vi "Launch Hardware Settings Dialog.vi"(8 "error in (no error)":errorcluster, 9 "Device":string, 10 "Msmt":string, 11 "Controller in":refnum<class "Controller.lvclass">) -> (0 "error out":errorcluster, 3 "Controller out":refnum<class "Controller.lvclass">)   [LabVIEW 2017, in "Controller Actor.lvlib" / "Controller.lvclass"]
uses:
  Controller.lvclass
  C:/Program Files (x86)/National Instruments/LabVIEW 2017/vi.lib/ActorFramework/Actor/Actor.lvclass
  Hardware/Hardware.lvclass/Hardware.ctl
  Hardware/HW Config/HW Configuration.lvclass/HW Configuration.ctl
  Controller.lvclass/Controller.ctl
  Hardware/HW Config/HW Configuration.lvclass
  <vilib>/ActorFramework/Actor/Actor.lvclass
  Hardware/Hardware.lvclass
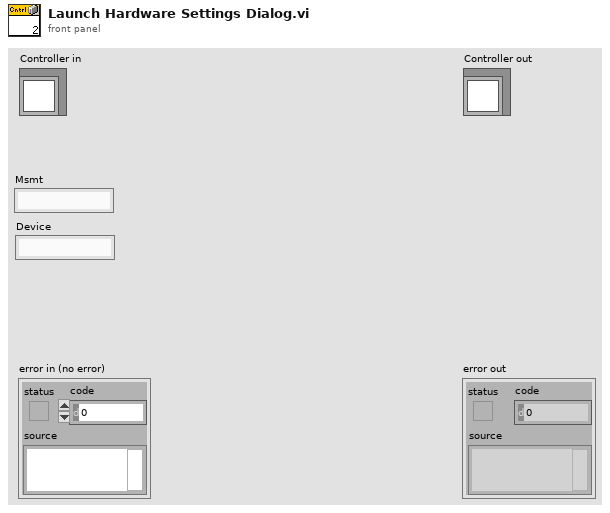
[diagram p1: front panel]
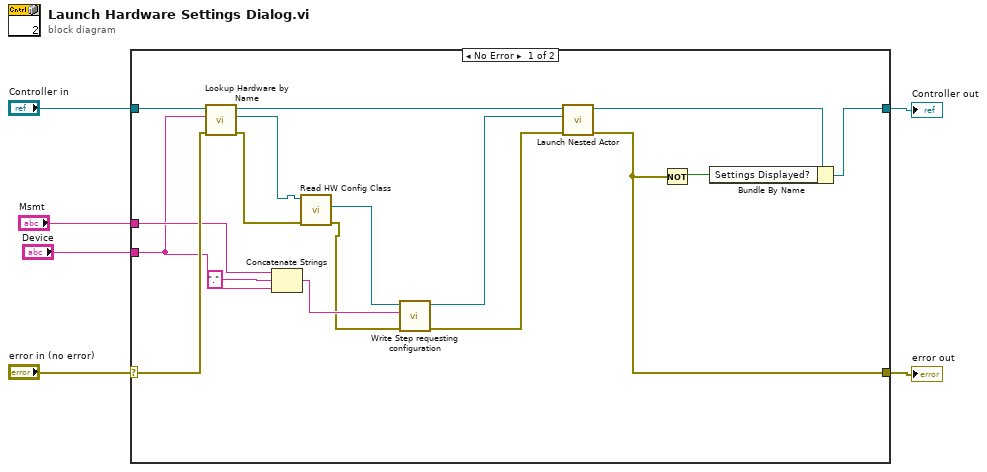
[diagram p0: block diagram]
diagram:
  n1 = case shown="No Error" "error in (no error)" {
    selector: "error in (no error)" -> [w20 w25]
    tunnel: [w16 w25] -> w5
    tunnel: [w22 w24] -> w3
    tunnel: "Controller in" -> [w21 w24]
    tunnel: "Device" -> [w14 _]
    tunnel: "Msmt" -> [w15 _]
    frame No Error {
      n2 = call "Lookup Hardware by Name.vi"("error in (no error)"=w20, "Device Name"=w14, "Controller in"=w21) -> ("error out"=w9:errorcluster, "Hardware.lvclass"=w10:refnum<class "Hardware.lvclass">, "Controller out"=w19:refnum<class "Controller.lvclass">)  [unwired: 6 in]
      n3 = Concatenate Strings(w15, "." ("string"), w14) -> (w12:string)
      n4 = call "Read HW Config Class.vi"("error in (no error)"=w9, "Hardware in"=w10) -> ("error out"=w8:errorcluster, "Hardware.lvlib:HW Configuration.lvclass"=w7:refnum<class "HW Configuration.lvclass">)  [unwired: 7 in, 1 out]
      n5 = call "Write Step requesting configuration.vi"("error in (no error)"=w8, "Step requesting configuration"=w12, "HW Configuration in"=w7) -> ("error out"=w17:errorcluster, "HW Configuration out"=w18:refnum<class "HW Configuration.lvclass">)  [unwired: 7 in]
      n6 = call <vilib>:"Launch Nested Actor.vi"("error in (no error)"=w17, "Nested Actor"=w18, "Caller Actor in"=w19) -> ("error out"=w16:errorcluster, "Caller Actor out"=w11:refnum<class "Controller.lvclass">)  [unwired: 6 in, 1 out]
      n7 = Not(x=w16) -> (.not. x?=w23:bool)
      n8 = Bundle By Name(cluster=w11, "Settings Displayed?"=w23) -> (w22:refnum<class "Controller.lvclass">)
    }
    frame Error {
    }
  }
  "error out" <- w5
  "Controller out" <- w3
